vi "com_inst.vi"(3 "Stop current":dbl format="%#_6p", 4 "Start current":dbl format="%#_6p", 5 "VISA session (for class)":refnum<visa-resource-name>) -> (0 "XTC":i32, 1 "SEN":i32, 2 "concatenated string":string)   [LabVIEW 2015]
doc: "This VI gets the initial parameters of the Lock-In by converting the number read into the valid string. We have two array of strings (for the sensitivity and time constant) where each index corresponds to the Lock-In number obtained by the commands \"SEN\" or \"XTC\" respectively."
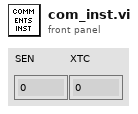
[diagram p1: front panel]
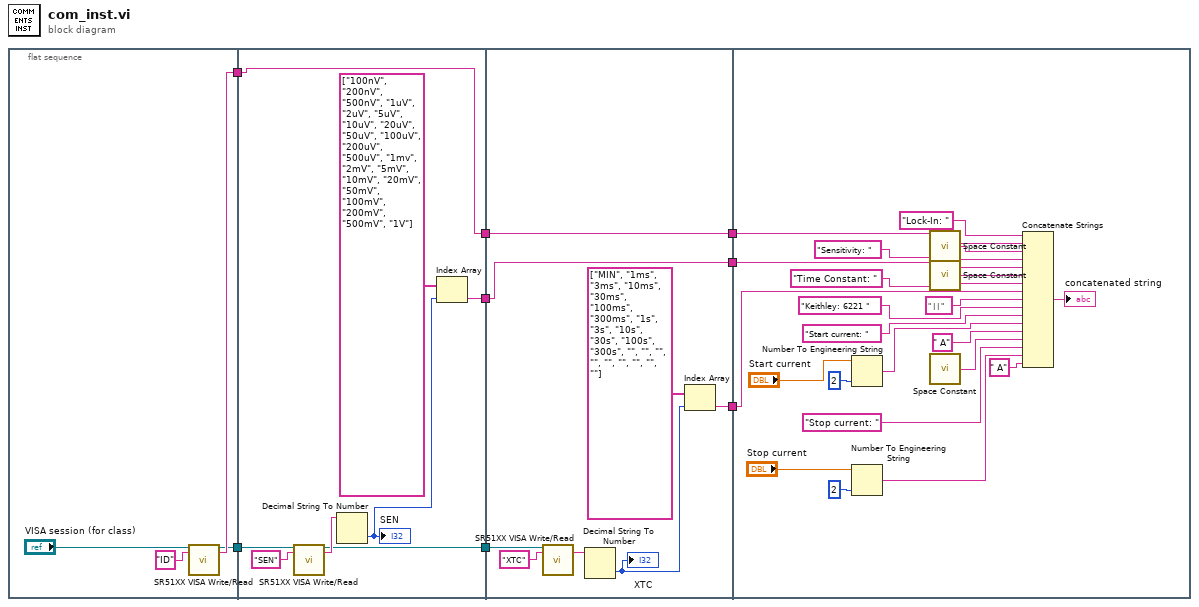
[diagram p0: block diagram]
diagram:
  n1 = flat-sequence {
    tunnel: [w10] -> w8
    tunnel: [w9] -> w7
    tunnel: [w17] -> w6
    tunnel: w8 -> [w16]
    tunnel: [w16] -> w4
    tunnel: w7 -> [w15]
    tunnel: [w14] -> w2
    tunnel: w6 -> [w28]
    tunnel: [w28] -> w5
    tunnel: w4 -> [w27]
    tunnel: [w27] -> w3
    tunnel: w2 -> [w25]
    tunnel: [w21] -> w1
    tunnel: w5 -> [w29]
    tunnel: w3 -> [w33]
    tunnel: w1 -> [w30]
    frame #0 {
      n2 = call "SR51XX VISA Write/Read"("VISA session (for class)"="VISA session (for class)", "Write Command String"="ID") -> ("VISA session"=w9:refnum<visa-resource-name>, "Response 1"=w10:string)  [unwired: 6 in, 10 out]
    }
    frame #1 {
      n3 = call "SR51XX VISA Write/Read"("VISA session (for class)"=w15, "Write Command String"="SEN") -> ("VISA session"=w14:refnum<visa-resource-name>, "Response 1"=w20:string)  [unwired: 6 in, 10 out]
      n4 = Decimal String To Number(string=w20) -> (number=w13:i32)  [unwired: 2 in, 1 out]
      "SEN" <- w13
      n5 = Index Array(array=string[] ["100nV", "200nV", "500nV", "1uV", "2uV", "5uV", "10uV", "20uV", "50uV", "100uV", "200uV", "500uV", "1mv", "2mV", "5mV", "10mV", "20mV", "50mV", "100mV", "200mV", "500mV", "1V"], index=w13) -> (element=w17:string)
    }
    frame #2 {
      n6 = call "SR51XX VISA Write/Read"("VISA session (for class)"=w25, "Write Command String"="XTC") -> ("Response 1"=w24:string)  [unwired: 6 in, 11 out]
      n7 = Decimal String To Number(string=w24) -> (number=w22:i32)  [unwired: 2 in, 1 out]
      "XTC" <- w22
      n8 = Index Array(array=string[] ["MIN", "1ms", "3ms", "10ms", "30ms", "100ms", "300ms", "1s", "3s", "10s", "30s", "100s", "300s", "", "", "", "", "", "", "", "", ""], index=w22) -> (element=w21:string)
    }
    frame #3 {
      n9 = Number To Engineering String(2:i16 2 ("precision (6)"), 4:"Start current") -> (0:w45:string)  [unwired: 2 in]
      n10 = Number To Engineering String(2:i16 2 ("precision (6)"), 4:"Stop current") -> (0:w49:string)  [unwired: 2 in]
      n11 = call <vilib>:"Space Constant.vi"() -> ("String"=w35:string)
      n12 = call <vilib>:"Space Constant.vi"() -> ("String"=w32:string)
      n13 = call <vilib>:"Space Constant.vi"() -> ("String"=w47:string)
      n14 = Concatenate Strings("Lock-In: " ("string"), w33, w35, "Sensitivity: " ("string"), w29, w32, "Time Constant: " ("string"), w30, " | | " ("string"), "Keithley: 6221 " ("string"), "Start current: " ("string"), w45, " A" ("string"), w47, "Stop current: " ("string"), w49, " A" ("string")) -> (→"concatenated string":string)
    }
  }
